vi "setLabels.vi"(7 "LabVIEW Web Service Request":refnum<class "Web Request.lvclass">) -> ()   [LabVIEW 2016]
uses:
  <vilib>/wsapi/Web Request.lvclass
  Typedef/MAC & Labels.ctl
  <vilib>/Utility/file.llb/Write Delimited Spreadsheet (string).vi
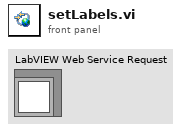
[diagram p1: front panel]
types:
  T1 = typedef "MAC & Labels.ctl" = cluster{"MAC list":string[], "Label list":string[]}
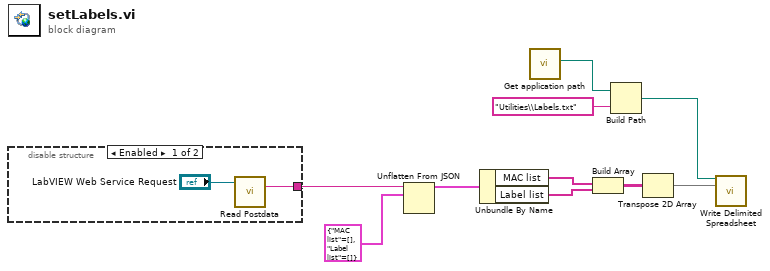
[diagram p0: block diagram]
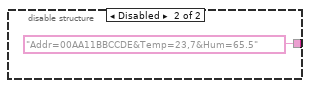
[diagram p2: hidden frame]
diagram:
  n1 = disable-structure shown="Enabled" {
    disable-tunnel: [w11 "Addr=00AA11BBCCDE&Temp=23,7&Hum=65.5" ("input string")] -> w9
    frame Enabled {
      n2 = call <vilib>:"Read Postdata.vi"("LabVIEW Web Service Request"="LabVIEW Web Service Request") -> ("postdata"=w11:string)  [unwired: 12 in, 2 out]
    }
    frame Disabled {
    }
  }
  n3 = Unflatten From JSON(JSON string=w9, type and defaults=T1 {"MAC list"=[], "Label list"=[]} ("MAC-label")) -> (value=w7:T1)  [unwired: 5 in, 1 out]
  n4 = Unbundle By Name(w7) -> ("MAC list"=w6:string[], "Label list"=w5:string[])
  n5 = call "Get application path.vi"() -> ("Application path"=w1:path)  [unwired: 11 in]
  n6 = Build Array(w6, w5) -> (w4:string[][])
  n7 = Build Path(base path=w1, name or relative path="Utilities\\Labels.txt") -> (appended path=w10:path)
  n8 = Transpose 2D Array(2D array=w4) -> (transposed array=w3:string[][])
  n9 = call-poly <vilib>:"Write Delimited Spreadsheet.vi"("file path (dialog if empty)"=w10, "2D data"=w3) -> ()  [unwired: 12 in, 2 out]
